vi "ITC503_Open_Queue.vi"(8 "error in (no error)":errorcluster) -> (0 "error out":errorcluster, 2 "queue out":refnum<queue>)   [LabVIEW 2019]
uses:
  ITC503/ITC503_control.ctl
  Global/Global Variables/Queues_global.vi
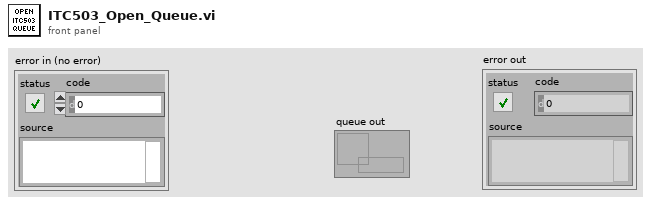
[diagram p1: front panel]
types:
  T1 = typedef "ITC503_control.ctl" = cluster{"Setpoint (K)":dbl, "Rate (K/min)":dbl, "Go to Set":bool, "Set Heater SP":bool, "Set NV SP":bool, "Change Heater Status":bool, "Change NV Status":bool, "Set Auto PID":bool, "Stopp":bool, "Control Channel":bool, "Heater SP":dbl, "NV Setpoint":dbl}
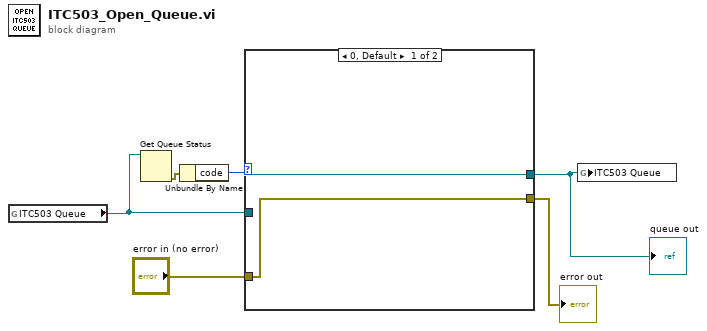
[diagram p0: block diagram]
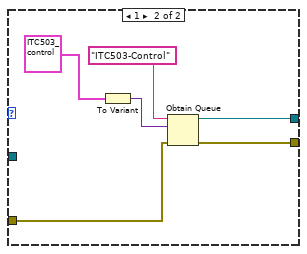
[diagram p2: hidden frame]
diagram:
  n1 = global read "Queues_global.vi" "ITC503 Queue"() -> (w4:refnum<queue>)
  n2 = Get Queue Status(queue=w4) -> (error out=w6:errorcluster)  [unwired: 2 in, 7 out]
  n3 = Unbundle By Name(w6) -> ("code"=w5:i32)
  n4 = case shown="0, Default" w5 {
    tunnel: w4 -> [w8 _]
    tunnel: [w8 w11] -> w3
    tunnel: "error in (no error)" -> [w7 w10]
    tunnel: [w7 w9] -> w1
    frame 0, Default {
    }
    frame 1 {
      n5 = To Variant(anything=T1 {"Setpoint (K)"=0.0, "Rate (K/min)"=3.4572, "Go to Set"=FALSE, "Set Heater SP"=FALSE, "Set NV SP"=FALSE, "Change Heater Status"=FALSE, "Change NV Status"=FALSE, "Set Auto PID"=FALSE, "Stopp"=FALSE, "Control Channel"=FALSE, "Heater SP"=0.0, "NV Setpoint"=0.0} ("ITC503-Control")) -> (Variant=w12:variant)
      n6 = Obtain Queue(name (unnamed)="ITC503-Control", element data type=w12, error in (no error)=w10) -> (queue out=w11:refnum<queue>, error out=w9:errorcluster)  [unwired: 2 in, 1 out]
    }
  }
  "queue out" <- w3
  "error out" <- w1
  n7 = global write "Queues_global.vi" "ITC503 Queue"(w3) -> ()
